vi "Write limit_y.vi"(8 "error in (no error)":errorcluster, 10 "limit_y":dbl, 11 "PongPanel in":refnum<class "PongPanel.lvclass">) -> (0 "error out":errorcluster, 3 "PongPanel out":refnum<class "PongPanel.lvclass">)   [LabVIEW 2019, in "RT_Game.lvlib" / "PongPanel.lvclass"]
uses:
  PongPanel.lvclass
  PongPanel.lvclass/PongPanel.ctl
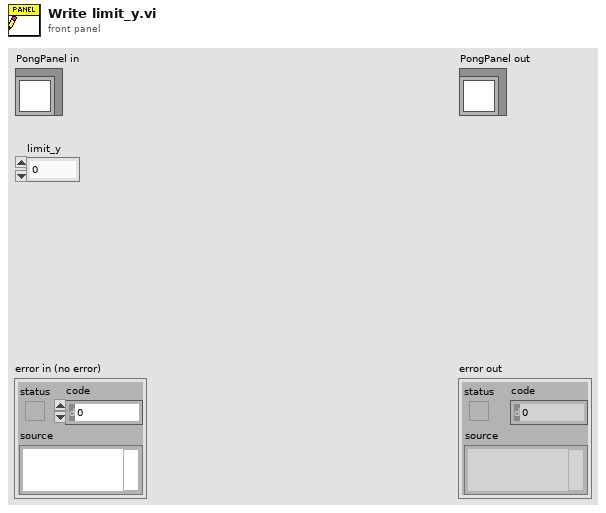
[diagram p1: front panel]
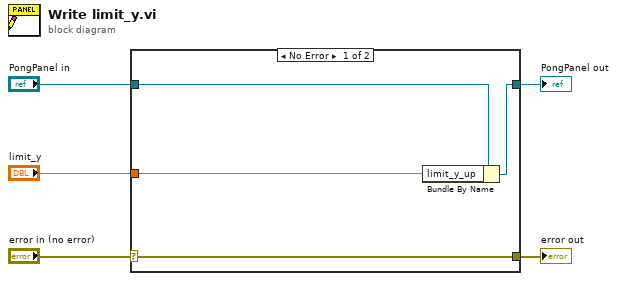
[diagram p0: block diagram]
diagram:
  n1 = case shown="No Error" "error in (no error)" {
    selector: "error in (no error)" -> [w9 w10]
    tunnel: [w9 w10] -> w4
    tunnel: [w7 w11] -> w2
    tunnel: "PongPanel in" -> [w8 w11]
    tunnel: "limit_y" -> [w6 _]
    frame No Error {
      n2 = Bundle By Name(cluster=w8, "limit_y_up"=w6) -> (w7:refnum<class "PongPanel.lvclass">)
    }
    frame Error {
    }
  }
  "error out" <- w4
  "PongPanel out" <- w2
